vi "SHT21.vi"() -> ()   [LabVIEW 2019]
uses:
  <vilib>/MakerHub/LINX/Public/Utilities/Open Local.vi
  SHT21_class/SHT21.lvclass
  <vilib>/MakerHub/LINX/LMH-LINX.lvlib
panel:
  out "RH":dbl(graph)
  out "Temp":dbl(graph)
  in  "stop":bool
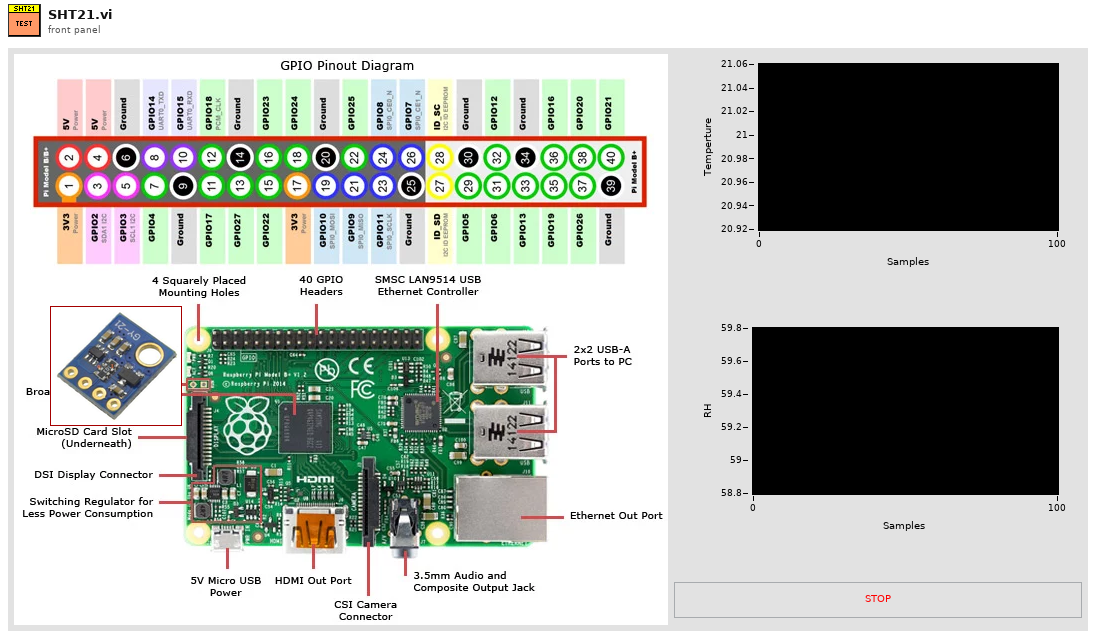
[diagram p1: front panel]
types:
  T1 = typedef "LMH-LINX.lvlib/LINX Ref.ctl" = cluster{"IO":T2, "Interface":T3, "LINX Device Config":T4}
  T2 = typedef "LMH-LINX.lvlib/Platform.ctl" = enum16{"Remote", "Local"}
  T3 = typedef "LMH-LINX.lvlib/Interface.ctl" = enum16{"Serial", "TCP"}
  T4 = typedef "LMH-LINX.lvlib/Device.lvlib/LINX Device Config.ctl" = cluster{"Interface":T3, "COM Port":refnum<visa-resource-name>, "TCP Configuration":T5, "Device Family":u8, "Device ID":u8, "Device Name":string, "TCP Ref":refnum<k5>, "Channels":T6}
  T5 = typedef "LMH-LINX.lvlib/Device.lvlib/TCP Config.ctl" = cluster{"IP Address":string, "Port":u16}
  T6 = typedef "LMH-LINX.lvlib/Channels.ctl" = cluster{"DI":u8[], "DO":u8[], "AI":u8[], "AO":u8[], "PWM":u8[], "QE":u8[], "UART":u8[], "I2C 2":u8[], "SPI":u8[], "CAN":u8[], "Servo":u8[], "AI Ref (V)":dbl, "AI Resolution (Bits)":u8, "AO Ref (V)":dbl, "AO Resolution (Bits)":u8}
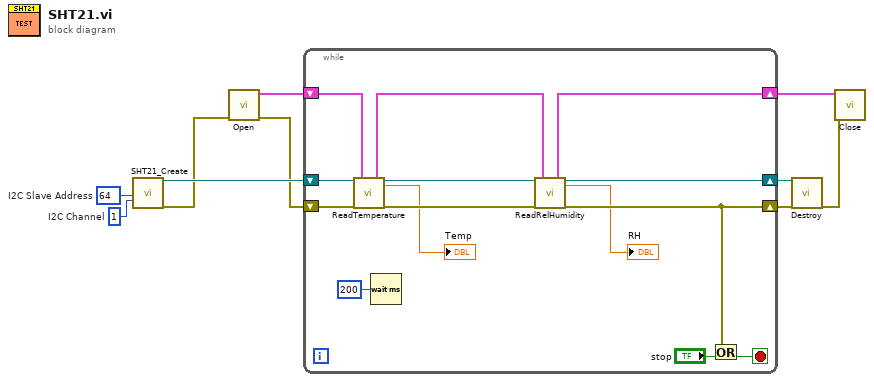
[diagram p0: block diagram]
diagram:
  w2 = u8 1  # I2C Channel
  w8 = u8 64  # I2C Slave Address
  n1 = call "SHT21_Create.vi"("I2C Slave Address (0)"=w8, "I2C Channel (0)"=w2) -> ("reference out"=w6:refnum<class "SHT21.lvclass">, "error out"=w1:errorcluster)  [unwired: 16 in]
  n2 = call-poly <vilib>:"Open.vi"("Error In"=w1) -> ("Error Out"=w3:errorcluster, "LINX Resource"=w4:T1)  [unwired: 8 in, 1 out]
  n3 = while {
    shift-right: [w15] -> w10
    shift-left: w6 -> [w22]
    shift-right: [w16] -> w9
    shift-left: w3 -> [w21]
    shift-right: [w13] -> w7
    shift-left: w4 -> [w20]
    stop <- w23 stop-if-true
    n4 = call-dynamic "ReadTemperature.vi"("reference in"=w22, "error in (no error)"=w21, "LINX Resource"=w20) -> ("LINX Resource"=w14:T1, "reference out"=w18:refnum<class "SHT21.lvclass">, "Temperature"=→"Temp":dbl, "error out"=w17:errorcluster)  [unwired: 12 in, 1 out]
    n5 = Wait (ms)(milliseconds to wait=u32 200) -> ()  [unwired: 1 out]
    n6 = call-dynamic "ReadRelHumidity.vi"("reference in"=w18, "error in (no error)"=w17, "LINX Resource"=w14) -> ("LINX Resource"=w13:T1, "reference out"=w15:refnum<class "SHT21.lvclass">, "RH"=→"RH":dbl, "error out"=w16:errorcluster)  [unwired: 12 in, 1 out]
    n7 = Or(x=w16, y="stop") -> (x .or. y?=w23:bool)
  }
  n8 = call-dynamic "Destroy.vi"("reference in"=w10, "error in (no error)"=w9) -> ("error out"=w5:errorcluster)  [unwired: 16 in, 1 out]
  n9 = call <vilib>:"Close.vi"("Error In"=w5, "LINX Resource"=w7) -> ()  [unwired: 9 in, 1 out]
